vi "Cymbal.vi"(11 "Trigger":bool) -> (3 "Cymbal Out":fxp<+/-,8,8>)   [LabVIEW 2015]
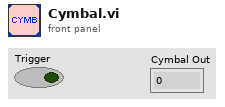
[diagram p1: front panel]
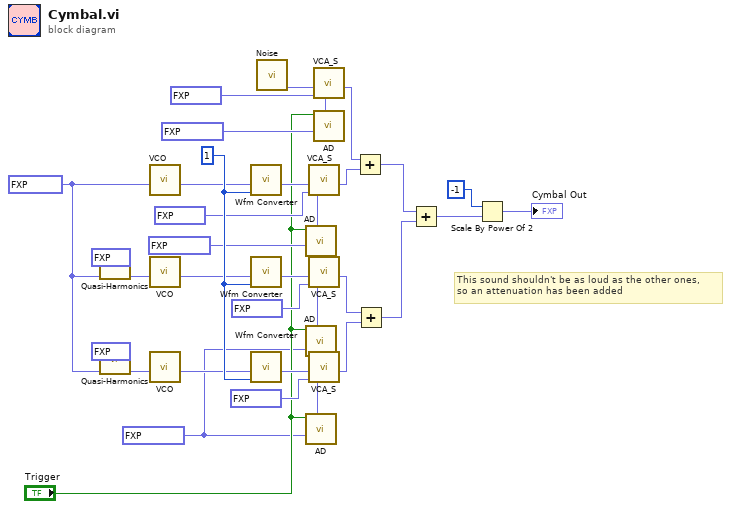
[diagram p0: block diagram]
diagram:
  w28 = u8 1 ("select")
  w1 = fxp<+,16,0> 4.57763671875e-05 ("Dec 4")
  w30 = fxp<+,32,32> 94489281.0 ("M")
  # "This sound shouldn't be as loud as the other ones,\nso an attenuation has been added"
  n1 = call "Quasi-Harmonics.vi"("Relative Freq"=fxp<+,8,3> 0.8125 ("relative f 3"), "1st partial"=w30) -> ("Result Partial"=w19:fxp<+,32,32>)  [unwired: 9 in]
  n2 = call "Quasi-Harmonics.vi"("Relative Freq"=fxp<+,8,3> 5.1875 ("relative f 4"), "1st partial"=w30) -> ("Result Partial"=w20:fxp<+,32,32>)  [unwired: 9 in]
  n3 = call "VCO.vi"("M"=w30) -> ("Sine Sample"=w16:fxp<+/-,8,8>)  [unwired: 10 in]
  n4 = call "VCO.vi"("M"=w19) -> ("Sine Sample"=w24:fxp<+/-,8,8>)  [unwired: 10 in]
  n5 = call "VCO.vi"("M"=w20) -> ("Sine Sample"=w26:fxp<+/-,8,8>)  [unwired: 10 in]
  n6 = call "Wfm Converter.vi"("Select"=w28, "Sample In"=w16) -> ("Sample Out"=w23:fxp<+/-,8,8>)  [unwired: 9 in]
  n7 = call "Wfm Converter.vi"("Select"=w28, "Sample In"=w24) -> ("Sample Out"=w25:fxp<+/-,8,8>)  [unwired: 9 in]
  n8 = call "Wfm Converter.vi"("Select"=w28, "Sample In"=w26) -> ("Sample Out"=w27:fxp<+/-,8,8>)  [unwired: 9 in]
  n9 = call "Noise.vi"() -> ("White Noise Out"=w29:fxp<+/-,8,8>)  [unwired: 11 in]
  n10 = call "AD.vi"("1/Decay"=fxp<+,16,0> 1.52587890625e-05 ("Dec"), "Trigger"="Trigger") -> ("Sample Out"=w5:fxp<+,8,0>)  [unwired: 9 in]
  n11 = call "AD.vi"("1/Decay"=w1, "Trigger"="Trigger") -> ("Sample Out"=w4:fxp<+,8,0>)  [unwired: 9 in]
  n12 = call "AD.vi"("1/Decay"=w1, "Trigger"="Trigger") -> ("Sample Out"=w2:fxp<+,8,0>)  [unwired: 9 in]
  n13 = call "VCA_S.vi"("EG"=w5, "Amount"=fxp<+,8,0> 0.99609375, "Sample In"=w23) -> ("Sample Out"=w33:fxp<+/-,8,8>)  [unwired: 8 in]
  n14 = call "VCA_S.vi"("EG"=w4, "Amount"=fxp<+,8,0> 0.30078125 ("Amount 3"), "Sample In"=w25) -> ("Sample Out"=w17:fxp<+/-,8,8>)  [unwired: 8 in]
  n15 = call "VCA_S.vi"("EG"=w2, "Amount"=fxp<+,8,0> 0.99609375 ("Amount 4"), "Sample In"=w27) -> ("Sample Out"=w18:fxp<+/-,8,8>)  [unwired: 8 in]
  n16 = call "AD.vi"("1/Decay"=fxp<+,16,0> 4.57763671875e-05 ("DecNoise"), "Trigger"="Trigger") -> ("Sample Out"=w7:fxp<+,8,0>)  [unwired: 9 in]
  n17 = call "VCA_S.vi"("EG"=w7, "Amount"=fxp<+,8,0> 0.99609375 ("Noise Amount"), "Sample In"=w29) -> ("Sample Out"=w32:fxp<+/-,8,8>)  [unwired: 8 in]
  n18 = Add(x=w32, y=w33) -> (x+y=w34:fxp<+/-,8,8>)
  n19 = Add(x=w17, y=w18) -> (x+y=w31:fxp<+/-,8,8>)
  n20 = Add(x=w34, y=w31) -> (x+y=w15:fxp<+/-,8,8>)
  n21 = Scale By Power Of 2(n=i16 -1, x=w15) -> (x*2^n=→"Cymbal Out":fxp<+/-,8,8>)
